vi "Update Current Pixel Locations.vi"() -> (3 "End of data?":bool)   [LabVIEW 2013]
doc: "Updates the current pixel locations for X and Y. Increments X position by 10. If row is complete, reset x position to 0 and increment Y. If X and Y are complete, reset position to 0,0."
uses:
  Globals/Pixel Location Global.vi
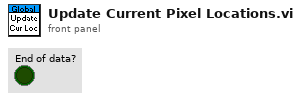
[diagram p1: front panel]
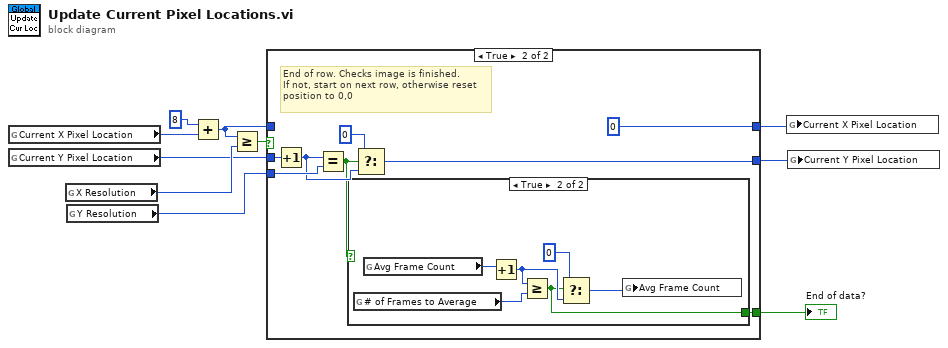
[diagram p0: block diagram]
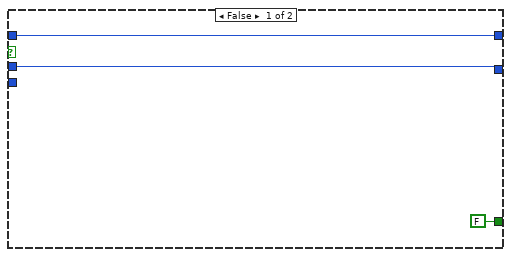
[diagram p2: hidden frame]
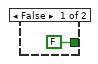
[diagram p3: hidden frame]
diagram:
  n1 = global read "Pixel Location Global.vi" "Current X Pixel Location"() -> (w8:u16)
  n2 = global read "Pixel Location Global.vi" "Current Y Pixel Location"() -> (w5:u16)
  n3 = global read "Pixel Location Global.vi" "X Resolution"() -> (w7:u16)
  n4 = global read "Pixel Location Global.vi" "Y Resolution"() -> (w4:u16)
  n5 = Add(x=u16 8, y=w8) -> (x+y=w3:u16)
  n6 = Greater Or Equal?(x=w3, y=w7) -> (x >= y?=w6:bool)
  n7 = case shown="True" w6 {
    tunnel: [w13 u16 0 ("Current X Pixel Location")] -> w2
    tunnel: w5 -> [w12 w20]
    tunnel: w4 -> [_ w19]
    tunnel: [w12 w15] -> w1
    tunnel: w3 -> [w13 _]
    tunnel: [FALSE w14] -> w10
    frame False {
    }
    frame True {
      # "End of row. Checks image is finished.\nIf not, start on next row, otherwise reset\nposition to 0,0"
      n8 = Increment(x=w20) -> (x+1=w17:u16)
      n9 = Equal?(x=w17, y=w19) -> (x = y?=w16:bool)
      n10 = case shown="True" w16 {
        tunnel: [FALSE w23] -> w14
        frame False {
        }
        frame True {
          n11 = global read "Pixel Location Global.vi" "# of Frames to Average"() -> (w27:u8)
          n12 = global read "Pixel Location Global.vi" "Avg Frame Count"() -> (w28:u8)
          n13 = Increment(x=w28) -> (x+1=w24:u8)
          n14 = Greater Or Equal?(x=w24, y=w27) -> (x >= y?=w23:bool)
          n15 = Select(t=u8 0 ("Frame Count"), s=w23, f=w24) -> (s? t:f=w26:u8)
          n16 = global write "Pixel Location Global.vi" "Avg Frame Count"(w26) -> ()
        }
      }
      n17 = Select(t=u16 0 ("Current X Pixel Location"), s=w16, f=w17) -> (s? t:f=w15:u16)
    }
  }
  "End of data?" <- w10
  n18 = global write "Pixel Location Global.vi" "Current X Pixel Location"(w2) -> ()
  n19 = global write "Pixel Location Global.vi" "Current Y Pixel Location"(w1) -> ()
